vi "Create gRPC Client.vi"(8 "error in (no error)":errorcluster, 10 "Data":T1={"Server Address"="localhost:50051", "Certificate Path"=""}, 11 "gRPC Client in":refnum<class "gRPC Client.lvclass">) -> (0 "error out":errorcluster, 3 "gRPC Client out":refnum<class "gRPC Client.lvclass">)   [LabVIEW 2019, in "gRPC Client (template.proto).lvlib" / "gRPC Client.lvclass"]
uses:
  gRPC Client.lvclass
  C:/Program Files (x86)/National Instruments/LabVIEW 2019/vi.lib/addons/_Workers/Library/Classes/Worker/Worker.lvclass
  rwr_Create gRPC Client.ctl
  gRPC Read/Initialization Data.ctl
  gRPC Read/Response Cases.ctl
  <vilib>/addons/_Workers/Library/Case Label.ctl
  <vilib>/gRPC/LabVIEW gRPC Library/Shared/grpcId.ctl
  rsp_Connection Notify.ctl
  gRPC Client.lvclass/gRPC Client.ctl
  gRPC Read/gRPC Read.lvclass
  Generated_client/Generated_client.lvlib
  <vilib>/gRPC/LabVIEW gRPC Library/grpc-lvsupport-release.lvlib
  <vilib>/addons/_Workers/Library/Workers.lvlib
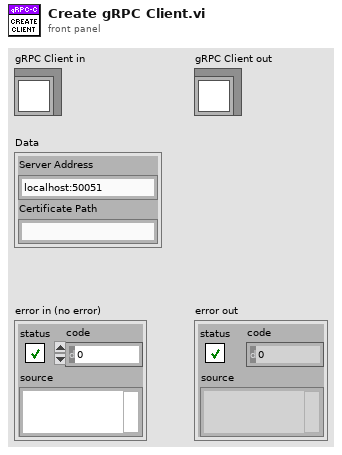
[diagram p1: front panel]
types:
  T1 = typedef "gRPC Client (template.proto).lvlib/gRPC Client.lvclass/rwr_Create gRPC Client.ctl" = cluster{"Server Address":string, "Certificate Path":string}
  T2 = typedef "gRPC Client (template.proto).lvlib/gRPC Client.lvclass/rsp_Connection Notify.ctl" = cluster{"gRPC ID":T3, "Connected?":bool}
  T3 = typedef "grpc-lvsupport-release.lvlib/grpcId.ctl" = u64
  T4 = typedef "gRPC Client (template.proto).lvlib/gRPC Read.lvclass/Initialization Data.ctl" = cluster{"Response Cases":T5, "Call ID":T3}
  T5 = typedef "gRPC Client (template.proto).lvlib/gRPC Read.lvclass/Response Cases.ctl" = cluster{"Receive Incoming gRPC Data":T6, "Connection Lost":T6}
  T6 = typedef "Workers.lvlib/Case Label.ctl" = string
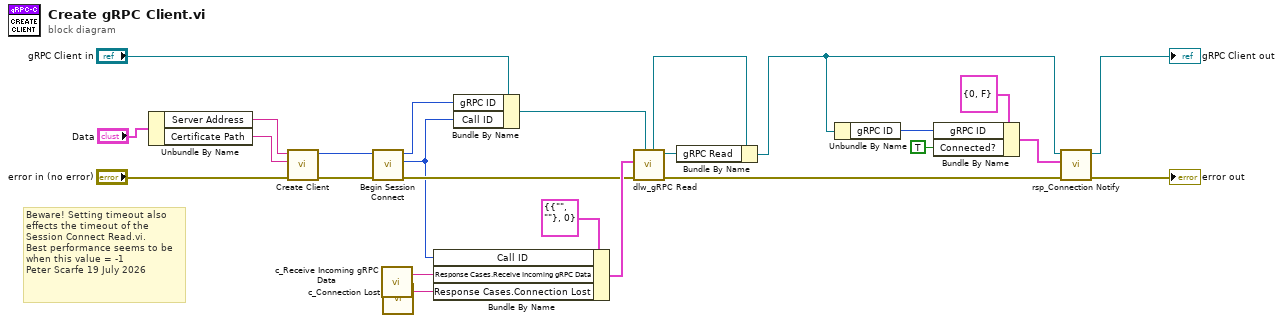
[diagram p0: block diagram]
diagram:
  # "Beware! Setting timeout also effects the timeout of the  Session Connect Read.vi.\nBest performance seems to be when this value = -1\nPeter Scarfe 19 July 2026"
  n1 = Unbundle By Name("Data") -> ("Server Address"=w20:string, "Certificate Path"=w19:string)
  n2 = call "Create Client.vi"("error in"="error in (no error)", "certificatePath"=w19, "address"=w20) -> ("error out"=w17:errorcluster, "gRPC ID Out"=w18:T3)  [unwired: 7 in]
  n3 = call "Begin Session Connect.vi"("error in"=w17, "gRPC ID"=w18) -> ("error out"=w14:errorcluster, "Call Id Out"=w9:T3, "gRPC ID out"=w10:T3)  [unwired: 7 in]
  n4 = call "c_Receive Incoming gRPC Data.vi"() -> ("Case Label"=w22:T6)  [unwired: 1 in]
  n5 = call "c_Connection Lost.vi"() -> ("Case Label"=w21:T6)  [unwired: 1 in]
  n6 = Bundle By Name(cluster=T4 {"Response Cases"={"Receive Incoming gRPC Data"="", "Connection Lost"=""}, "Call ID"=0} ("Initialization Data"), "Call ID"=w9, "Response Cases.Receive Incoming gRPC Data"=w22, "Response Cases.Connection Lost"=w21) -> (w23:T4)
  n7 = Bundle By Name(cluster="gRPC Client in", "gRPC ID"=w10, "Call ID"=w9) -> (w11:refnum<class "gRPC Client.lvclass">)
  n8 = call "dlw_gRPC Read.vi"("Caller in"=w11, "error in"=w14, "Initialization Data"=w23) -> ("error out"=w4:errorcluster, "gRPC Read out"=w25:refnum<class "gRPC Read.lvclass">, "dup Caller out"=w13:refnum<class "gRPC Client.lvclass">)  [unwired: 6 in]
  n9 = Bundle By Name(cluster=w13, "gRPC Read"=w25) -> (w2:refnum<class "gRPC Client.lvclass">)
  n10 = Unbundle By Name(w2) -> ("gRPC ID"=w1:T3)
  n11 = Bundle By Name(cluster=T2 {"gRPC ID"=0, "Connected?"=FALSE} ("Data in"), "gRPC ID"=w1, "Connected?"=TRUE) -> (w6:T2)
  n12 = call "rsp_Connection Notify.vi"("error in"=w4, "Data in"=w6, "gRPC Client in"=w2) -> ("error out"=→"error out":errorcluster, "dup gRPC Client out"=→"gRPC Client out":refnum<class "gRPC Client.lvclass">)  [unwired: 7 in]
